vi "test_variance_map_filtered _M_stripped.vi"() -> ()   [LabVIEW 2009]
doc: "Copyright (C) 2009, Stepan A. Baranov\nweb: http://www.OCTLab.org/\nemail: stepan@baranov.su"
uses:
  <vilib>/Analysis/NI_AALBase.lvlib
  OCTLib.dll
panel:
  out "min":dbl format="%0.2f"
  out "max":dbl format="%0.2f"
  out "offset":i32
  out "error out":errorcluster
  out "strip size":i32
  out "width":i32
  out "height":i32
  in  "Small/Big":bool
  out "loop #":i32
  out "RSM_STAT time":u32
  out "LabView time":u32
  out "RSM_STAT Array":dbl[][](array[numeric])
  out "LabView Array":dbl[][](array[numeric])
  in  "stop":bool
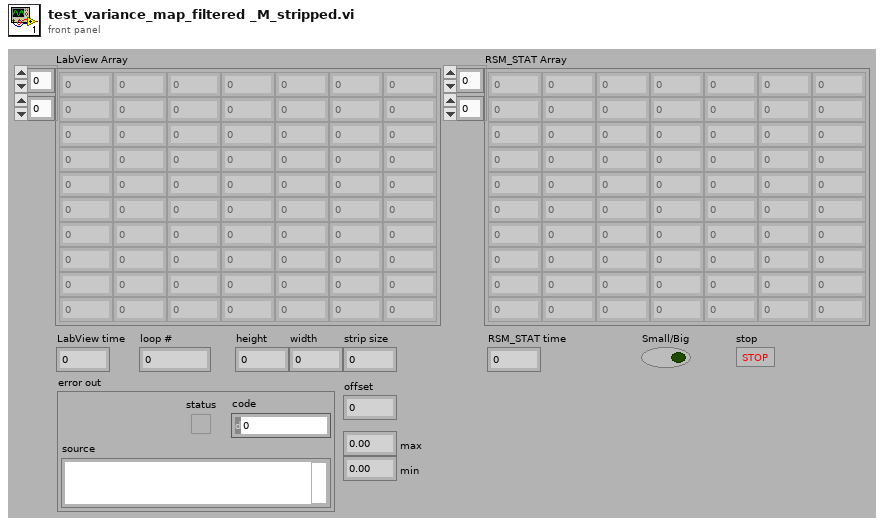
[diagram p1: front panel]
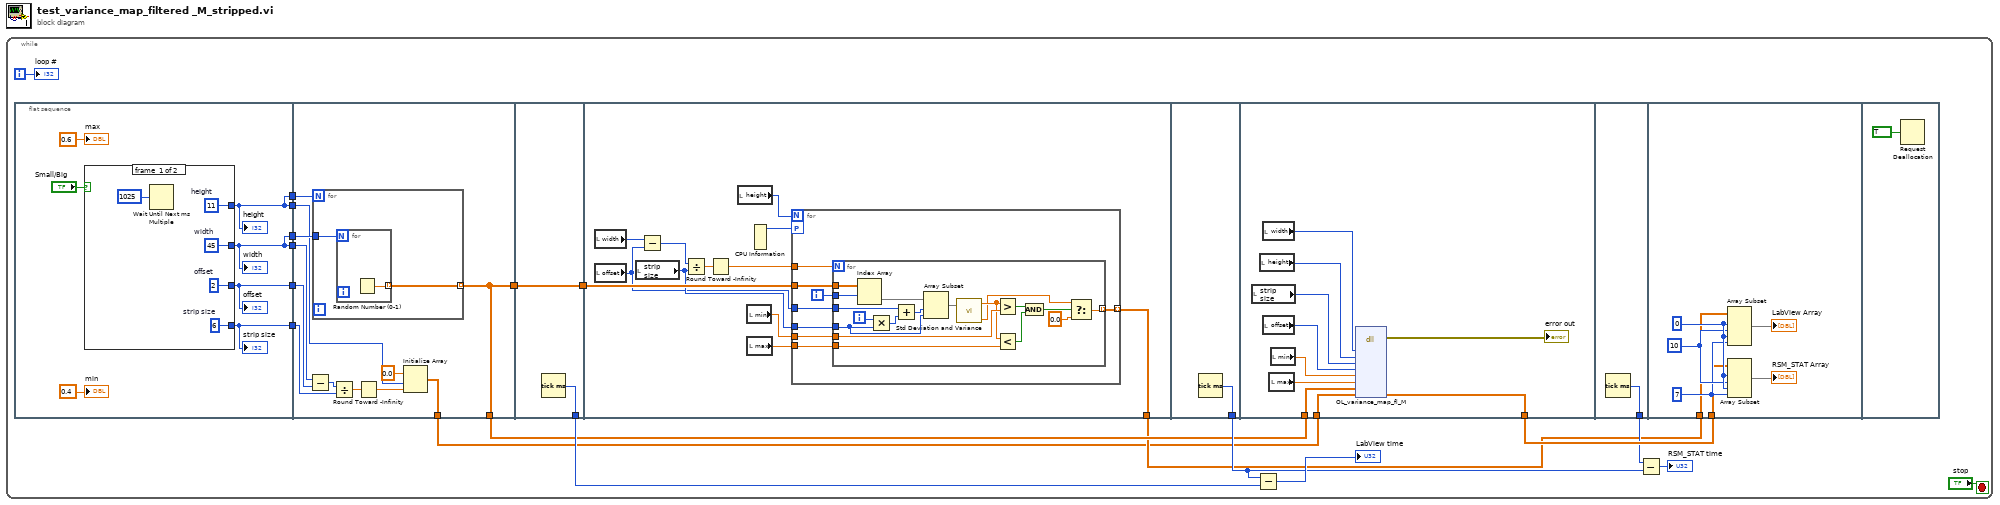
[diagram p0: block diagram]
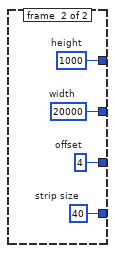
[diagram p2: hidden frame]
diagram:
  n1 = while {
    i -> [w12]
    stop <- "stop" stop-if-true
    n2 = flat-sequence {
      tunnel: [w23] -> w8
      tunnel: [w24] -> w7
      tunnel: [w25] -> w5
      tunnel: [w24] -> w4
      tunnel: [w23] -> w3
      tunnel: [w22] -> w1
      tunnel: [w45] -> w11
      tunnel: [w45] -> w9
      tunnel: w8 -> [w47]
      tunnel: w7 -> [w46]
      tunnel: w5 -> [w38]
      tunnel: w4 -> [w42]
      tunnel: w3 -> [w41]
      tunnel: [w43] -> w2
      tunnel: w1 -> [w40]
      tunnel: [w52] -> w17
      tunnel: [w51] -> w10
      tunnel: w9 -> [w51]
      tunnel: w10 -> [w64]
      tunnel: [w63] -> w6
      tunnel: [w91] -> w14
      tunnel: w11 -> [w100]
      tunnel: [w99] -> w18
      tunnel: w2 -> [w101]
      tunnel: [w102] -> w15
      tunnel: w18 -> [w105]
      tunnel: w6 -> [w104]
      frame #0 {
        n3 = case shown="True" "Small/Big" {
          tunnel: [w29 w35] -> w24
          tunnel: [w30 w34] -> w23
          tunnel: [w31 w33] -> w25
          tunnel: [w27 w32] -> w22
          frame #0 {
            w27 = 2  # offset
            w31 = 6  # strip size
            w30 = 45  # width
            w29 = 11  # height
            n4 = Wait Until Next ms Multiple(millisecond multiple=u32 1025) -> ()  [unwired: 1 out]
          }
          frame #1 {
            w32 = 4  # offset
            w33 = 40  # strip size
            w34 = 20000  # width
            w35 = 1000  # height
          }
        }
        "height" <- w24
        "width" <- w23
        "strip size" <- w25
        "offset" <- w22
        "max" <- 0.6 ("max")
        "min" <- 0.4 ("min")
      }
      frame #1 {
        n5 = Subtract(x=w41, y=w40) -> (x-y=w39:i32)
        n6 = for {
          N: w46 -> [_]
          tunnel: w47 -> [w49]
          tunnel: [w48] -> w45 mode=indexing
          n7 = for {
            N: w49 -> [_]
            tunnel: [w50] -> w48 mode=indexing
            n8 = Random Number (0-1)() -> (number: 0 to 1=w50:dbl)
          }
        }
        n9 = Divide(x=w39, y=w38) -> (x/y=w37:dbl)
        n10 = Round Toward -Infinity(1:w37) -> (0:w36:dbl)
        n11 = Initialize Array(0.0 ("element"), w42, w36) -> (w43:dbl[][])
      }
      frame #2 {
        n12 = Tick Count (ms)() -> (millisecond timer value=w52:u32)
      }
      frame #3 {
        n13 = local read "width"() -> (w62:i32)
        n14 = local read "offset"() -> (w53:i32)
        n15 = local read "strip size"() -> (w56:i32)
        n16 = Subtract(x=w62, y=w53) -> (x-y=w57:i32)
        n17 = Divide(x=w57, y=w56) -> (x/y=w55:dbl)
        n18 = Round Toward -Infinity(1:w55) -> (0:w54:dbl)
        n19 = local read "height"() -> (w58:i32)
        n20 = local read "min"() -> (w60:dbl)
        n21 = local read "max"() -> (w59:dbl)
        n22 = CPU Information() -> (4:w61:i32)  [unwired: 3 out]
        n23 = for {
          N: w58 -> [_]
          tunnel: w64 -> [w71]
          tunnel: [w70] -> w63 mode=indexing
          tunnel: w56 -> [w69]
          tunnel: w54 -> [w68]
          workers-P: w61 -> [_]
          tunnel: w60 -> [w67]
          tunnel: w59 -> [w66]
          tunnel: w53 -> [w65]
          i -> [w72]
          n24 = for {
            N: w68 -> [_]
            tunnel: w72 -> [w78]
            tunnel: w71 -> [w79]
            tunnel: [w85] -> w70 mode=indexing
            tunnel: w69 -> [w75]
            tunnel: w67 -> [w90]
            tunnel: w66 -> [w89]
            tunnel: w65 -> [w80]
            i -> [w82]
            n25 = Index Array(array=w79, index (row)=w78) -> (element=w77:dbl[])  [unwired: 1 in]
            n26 = Multiply(x=w82, y=w75) -> (x*y=w81:i32)
            n27 = Add(x=w80, y=w81) -> (x+y=w76:i32)
            n28 = Array Subset(array=w77, index=w76, length=w75) -> (w74:dbl[])
            n29 = call <vilib>:"Std Deviation and Variance.vi"("X"=w74) -> ("mean"=w83:dbl, "variance"=w73:dbl)  [unwired: 1 in, 1 out]
            n30 = Greater?(x=w83, y=w90) -> (0:w87:bool)
            n31 = Less?(x=w83, y=w89) -> (x < y?=w88:bool)
            n32 = And(x=w87, y=w88) -> (x .and. y?=w86:bool)
            n33 = Select(t=w73, s=w86, f=0.0) -> (s? t:f=w85:dbl)
          }
        }
      }
      frame #4 {
        n34 = Tick Count (ms)() -> (millisecond timer value=w91:u32)
      }
      frame #5 {
        n35 = local read "strip size"() -> (w95:i32)
        n36 = local read "height"() -> (w97:i32)
        n37 = local read "width"() -> (w98:i32)
        n38 = local read "offset"() -> (w94:i32)
        n39 = local read "max"() -> (w92:dbl)
        n40 = local read "min"() -> (w93:dbl)
        n41 = dll-call lib="OCTLib.dll" fn="OL_variance_map_fl_M"("width"=w98, "height"=w97, "stripsize"=w95, "offset"=w94, "min"=w93, "max"=w92, "input"=w100, "output"=w101) -> (error out=→"error out":errorcluster, "output"=w99:dbl[][])  [unwired: 11 in, 1 out]
      }
      frame #6 {
        n42 = Tick Count (ms)() -> (millisecond timer value=w102:u32)
      }
      frame #7 {
        w108 = 10 ("length")
        w107 = 7 ("length")
        w109 = 0 ("index")
        n43 = Array Subset(array=w104, index (row)=w109, length (row)=w108, index (col)=w109, length (col)=w107) -> (→"LabView Array":dbl[][])
        n44 = Array Subset(array=w105, index (row)=w109, length (row)=w108, index (col)=w109, length (col)=w107) -> (→"RSM_STAT Array":dbl[][])
      }
      frame #8 {
        n45 = Request Deallocation(TRUE ("flag")) -> ()
      }
    }
    n46 = Subtract(x=w14, y=w17) -> (x-y=→"LabView time":u32)
    n47 = Subtract(x=w15, y=w14) -> (x-y=→"RSM_STAT time":u32)
    "loop #" <- w12
  }
